vi "ARCO Main Server.vi"() -> ()   [LabVIEW 2017]
uses:
  <vilib>/OPCUA/controls/Data Type.ctl
  <vilib>/OPCUA/controls/Supported Security Policies.ctl
  <vilib>/OPCUA/server/Read Bool Array.vi
  <vilib>/OPCUA/NI OPC UA Server.lvlib
  <vilib>/OPCUA/NI OPC UA Utility.lvlib
panel:
  out "BoP Output Node":string
  out "BoP Input Node":string
  out "Result Boolean Control Node":string
  out "Result Numeric Control Node":string
  out "Result Data Node":string
  out "Spoof Boolean Control Node":string
  out "Spoof Numeric Control Node":string
  out "Spoof Data Node":string
  out "Chat Node":string
  out "Boolean Control Action Node":string
  out "Numeric Control Action Node":string
  out "certificate path 2":path
  out "certificate path":path
  out "error out":errorcluster
  out "CIET Data Node":string
  out "server endpoint URL":string
  in  "Stop":bool
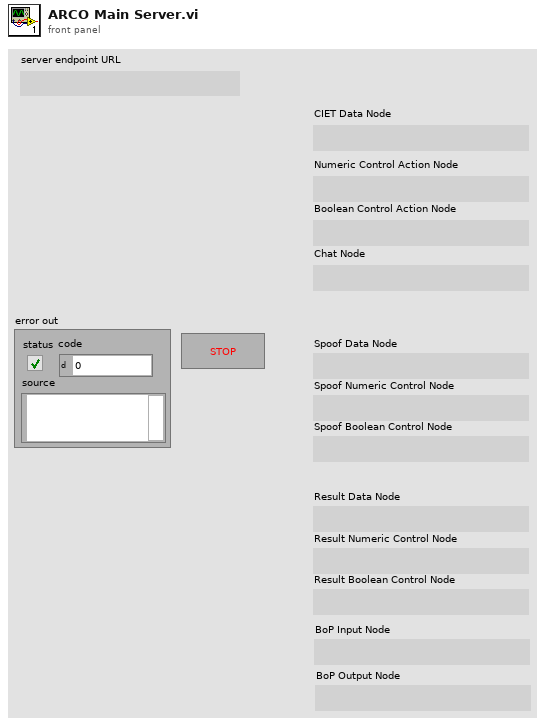
[diagram p1: front panel]
types:
  T1 = typedef "Data Type.ctl" = u16
  T2 = cluster{"name":string, "data type":T1, "access level":u16, "description":string}
  T3 = cluster{"name":string, "data type":T1, "access level 2":u16, "description":string}
  T4 = typedef "Supported Security Policies.ctl" = cluster{"None":bool, "Sign with Basic128Rsa15":bool, "Sign and Encrypt with Basic128Rsa15":bool, "Sign with Basic256":bool, "Sign and Encrypt with Basic256":bool}
  T5 = typedef "OPC UA Server Refnum.ctl" = refnum<k21>
  T6 = typedef "NodeId.ctl" = string
  T7 = cluster{"value[0]":bool, "value[1]":bool, "value[2]":bool, "value[3]":bool, "value[4]":bool, "value[5]":bool, "value[6]":bool, "value[7]":bool, "value[8]":bool}
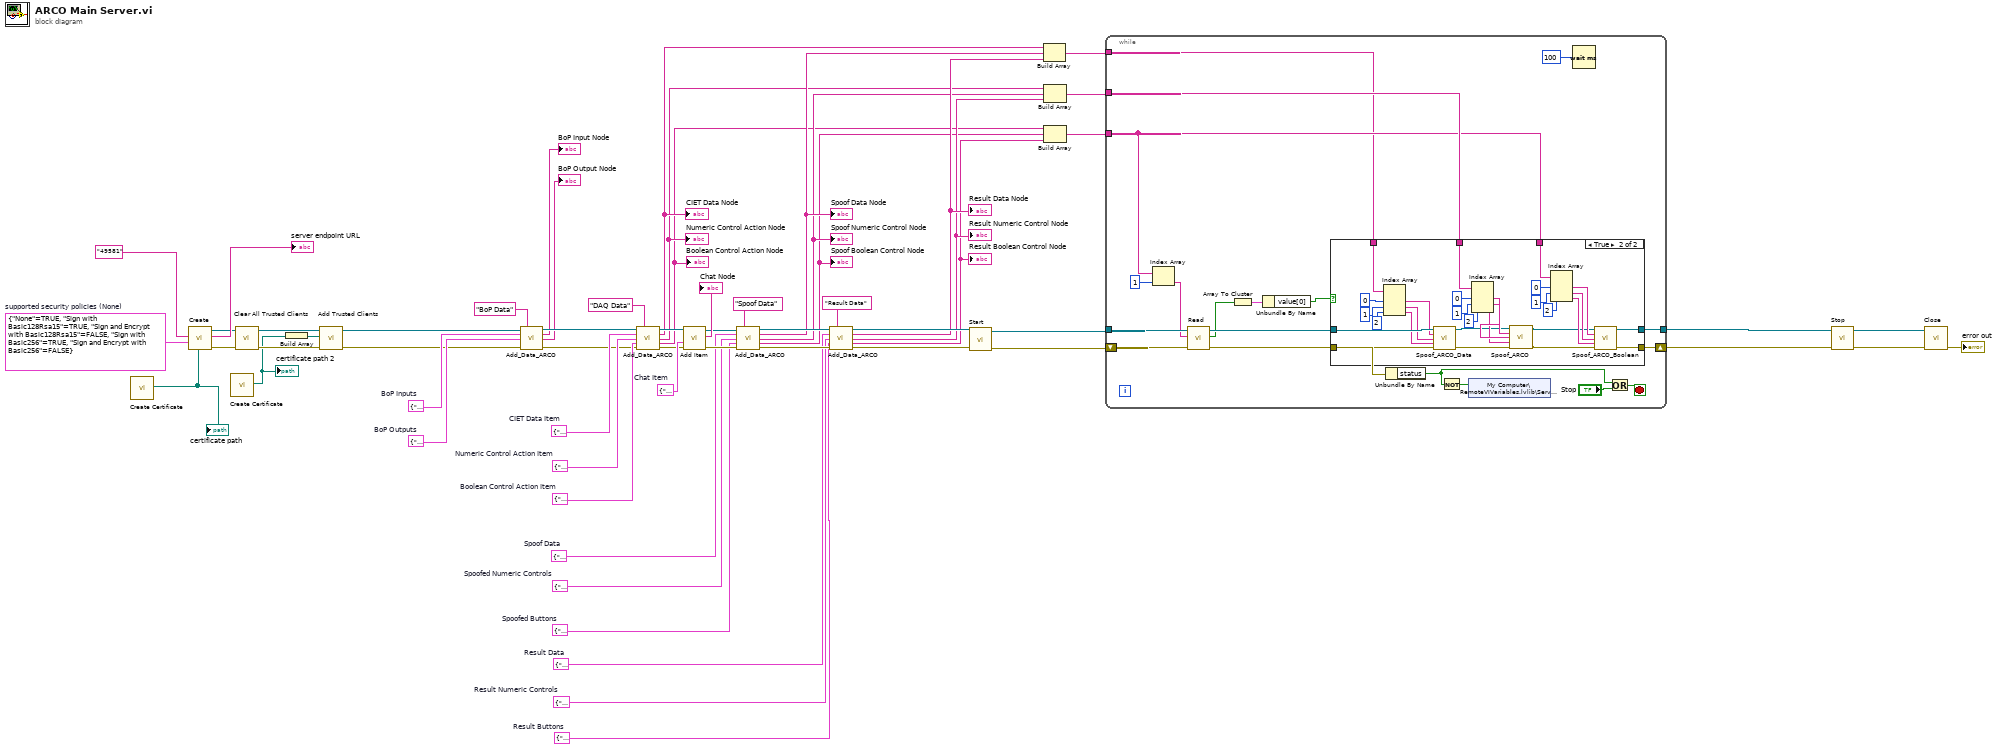
[diagram p0: block diagram]
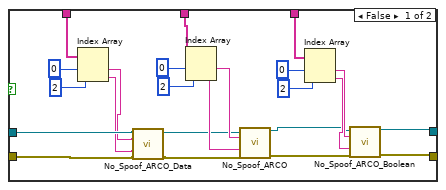
[diagram p2: hidden frame]
diagram:
  w7 = T2 {"name"="BoP Outputs", "data type"=111, "access level"=3, "description"="BoP Output Values"}  # BoP Outputs
  w8 = T2 {"name"="BoP Inputs", "data type"=111, "access level"=3, "description"="BoP Input Values"}  # BoP Inputs
  w25 = T2 {"name"="Spoofed Numeric Controls", "data type"=111, "access level"=3, "description"="Spoofed Setpoints"}  # Spoofed Numeric Controls
  w26 = T2 {"name"="Spoofed CIET Data", "data type"=111, "access level"=3, "description"="Spoofed CIET TC and FM"}  # Spoof Data
  w31 = T2 {"name"="Result Boolean Controls", "data type"=101, "access level"=3, "description"="Result Buttons"}  # Result Buttons
  w32 = T2 {"name"="Result Numeric Controls", "data type"=111, "access level"=3, "description"="Result Setpoints"}  # Result Numeric Controls
  w33 = T3 {"name"="Result CIET Data", "data type"=111, "access level 2"=3, "description"="Result CIET TC and FM"}  # Result Data
  w24 = T2 {"name"="Spoofed Boolean Controls", "data type"=101, "access level"=3, "description"="Spoofed Buttons"}  # Spoofed Buttons
  w45 = T2 {"name"="Chat", "data type"=12, "access level"=3, "description"="Chat"}  # Chat Item
  w41 = T2 {"name"="Boolean Control Actions", "data type"=101, "access level"=3, "description"="Buttons"}  # Boolean Control Action Item
  w42 = T2 {"name"="Numeric Control Actions", "data type"=111, "access level"=3, "description"="Setpoints"}  # Numeric Control Action Item
  w54 = T4 {"None"=TRUE, "Sign with Basic128Rsa15"=TRUE, "Sign and Encrypt with Basic128Rsa15"=FALSE, "Sign with Basic256"=TRUE, "Sign and Encrypt with Basic256"=FALSE}  # supported security policies (None)
  w43 = T2 {"name"="CIET Data", "data type"=111, "access level"=3, "description"="CIET TC and FM"}  # CIET Data Item
  n1 = call <vilib>:"Create Certificate.vi"() -> ("certificate path"=w49:path)  [unwired: 8 in, 3 out]
  "certificate path" <- w49
  n2 = call <vilib>:"Create.vi"("server certificate file"=w49, "supported security policies (None)"=w54, "TCP port (49580)"="49581") -> ("error out"=w50:errorcluster, "server endpoint URL"=→"server endpoint URL":string, "OPC UA server refnum out"=w51:T5)  [unwired: 6 in]
  n3 = call <vilib>:"Create Certificate.vi"() -> ("certificate path"=w48:path)  [unwired: 8 in, 3 out]
  "certificate path 2" <- w48
  n4 = call <vilib>:"Clear All Trusted Clients.vi"("error in (no error)"=w50, "OPC UA server refnum in"=w51) -> ("error out"=w52:errorcluster, "OPC UA server refnum out"=w53:T5)  [unwired: 8 in]
  n5 = Build Array(w48) -> (w47:path[])
  n6 = call <vilib>:"Add Trusted Clients.vi"("error in (no error)"=w52, "trusted client certificates"=w47, "OPC UA server refnum in"=w53) -> ("error out"=w5:errorcluster, "OPC UA server refnum out"=w6:T5)  [unwired: 7 in]
  n7 = call "Add_Data_ARCO.vi"("Refnum in"=w6, "folder name"="BoP Data", "item 1"=w8, "item 2"=w7, "error in (no error)"=w5) -> ("Refnum out"=w3:T5, "item node ID 1"=→"BoP Input Node":string, "item node ID 2"=→"BoP Output Node":string, "error out"=w4:errorcluster)  [unwired: 6 in, 1 out]
  n8 = call "Add_Data_ARCO.vi"("Refnum in"=w3, "folder name"="DAQ Data", "item 1"=w43, "item 2"=w42, "item 3"=w41, "error in (no error)"=w4) -> ("Refnum out"=w40:T5, "item node ID 1"=w20:string, "item node ID 2"=w17:string, "item node ID 3"=w14:string, "error out"=w39:errorcluster)  [unwired: 5 in]
  "CIET Data Node" <- w20
  "Numeric Control Action Node" <- w17
  "Boolean Control Action Node" <- w14
  n9 = call <vilib>:"Add Item.vi"("error in (no error)"=w39, "item"=w45, "OPC UA server refnum in"=w40) -> ("error out"=w36:errorcluster, "item node ID"=→"Chat Node":T6, "OPC UA server refnum out"=w37:T5)  [unwired: 4 in, 1 out]
  n10 = call "Add_Data_ARCO.vi"("Refnum in"=w37, "folder name"="Spoof Data", "item 1"=w26, "item 2"=w25, "item 3"=w24, "error in (no error)"=w36) -> ("Refnum out"=w34:T5, "item node ID 1"=w19:string, "item node ID 2"=w16:string, "item node ID 3"=w13:string, "error out"=w35:errorcluster)  [unwired: 5 in]
  "Spoof Data Node" <- w19
  "Spoof Numeric Control Node" <- w16
  "Spoof Boolean Control Node" <- w13
  n11 = call "Add_Data_ARCO.vi"("Refnum in"=w34, "folder name"="Result Data", "item 1"=w33, "item 2"=w32, "item 3"=w31, "error in (no error)"=w35) -> ("Refnum out"=w27:T5, "item node ID 1"=w18:string, "item node ID 2"=w15:string, "item node ID 3"=w12:string, "error out"=w28:errorcluster)  [unwired: 5 in]
  "Result Data Node" <- w18
  "Result Numeric Control Node" <- w15
  "Result Boolean Control Node" <- w12
  n12 = call <vilib>:"Start.vi"("error in (no error)"=w28, "OPC UA server refnum in"=w27) -> ("error out"=w11:errorcluster, "OPC UA server refnum out"=w59:T5)  [unwired: 7 in, 1 out]
  n13 = Build Array(w20, w19, w18) -> (w23:string[])
  n14 = Build Array(w17, w16, w15) -> (w22:string[])
  n15 = Build Array(w14, w13, w12) -> (w21:string[])
  n16 = while {
    tunnel: [w78] -> w58
    tunnel: w59 -> [w71]
    tunnel: w23 -> [w61]
    tunnel: w22 -> [w67]
    tunnel: w21 -> [w62]
    shift-right: [w76] -> w10
    shift-left: w11 -> [w72]
    stop <- w75 stop-if-true
    n17 = Index Array(array=w62, index=1) -> (element=w66:string)
    n18 = call-poly <vilib>:"Read.vi"("error in (no error)"=w72, "node ID"=w66, "OPC UA server refnum in"=w71) -> ("error out"=w69:errorcluster, "value"=w65:bool[], "OPC UA server refnum out"=w70:T5)  [unwired: 4 in, 2 out]
    n19 = Array To Cluster(array=w65) -> (cluster=w64:T7)
    n20 = Unbundle By Name(w64) -> ("value[0]"=w63:bool)
    n21 = case shown="True" w63 {
      tunnel: [w88 w131] -> w78
      tunnel: w70 -> [w82 w106]
      tunnel: w67 -> [w91 w118]
      tunnel: w62 -> [w96 w117]
      tunnel: [w87 w116] -> w76
      tunnel: w69 -> [w83 w107]
      tunnel: w61 -> [w86 w110]
      frame False {
        n22 = Index Array(array=w86, index #1=0, index #2=2 ("index")) -> (element #1=w81:string, element #2=w80:string)
        n23 = call "No_Spoof_ARCO_Data.vi"("OPC UA server refnum in"=w82, "DAQ Node"=w81, "Result Node"=w80, "error in (no error)"=w83) -> ("OPC UA server refnum out"=w85:T5, "error out"=w84:errorcluster)  [unwired: 10 in]
        n24 = Index Array(array=w91, index #1=0, index #2=2 ("index")) -> (element #1=w93:string, element #2=w92:string)
        n25 = call "No_Spoof_ARCO.vi"("OPC UA server refnum in"=w85, "DAQ Node"=w93, "Result Node"=w92, "error in (no error)"=w84) -> ("OPC UA server refnum out"=w90:T5, "error out"=w89:errorcluster)  [unwired: 10 in]
        n26 = Index Array(array=w96, index #1=0, index #2=2 ("index")) -> (element #1=w98:string, element #2=w97:string)
        n27 = call "No_Spoof_ARCO_Boolean.vi"("OPC UA server refnum in"=w90, "DAQ Node"=w98, "Result Node"=w97, "error in (no error)"=w89) -> ("OPC UA server refnum out"=w88:T5, "error out"=w87:errorcluster)  [unwired: 10 in]
      }
      frame True {
        n28 = Index Array(array=w110, index #1=0, index #2=1, index #3=2) -> (element #1=w103:string, element #2=w104:string, element #3=w105:string)
        n29 = call "Spoof_ARCO_Data.vi"("OPC UA server refnum in"=w106, "DAQ Node"=w103, "Spoof Node"=w104, "Result Node"=w105, "error in (no error)"=w107) -> ("OPC UA server refnum out"=w109:T5, "error out"=w108:errorcluster)  [unwired: 9 in]
        n30 = Index Array(array=w118, index #1=0, index #2=1, index #3=2) -> (element #1=w115:string, element #2=w114:string, element #3=w113:string)
        n31 = call "Spoof_ARCO.vi"("OPC UA server refnum in"=w109, "DAQ Node"=w115, "Spoof Node"=w114, "Result Node"=w113, "error in (no error)"=w108) -> ("OPC UA server refnum out"=w112:T5, "error out"=w111:errorcluster)  [unwired: 9 in]
        n32 = Index Array(array=w117, index #1=0, index #2=1, index #3=2) -> (element #1=w119:string, element #2=w120:string, element #3=w121:string)
        n33 = call "Spoof_ARCO_Boolean.vi"("OPC UA server refnum in"=w112, "DAQ Node"=w119, "Spoof Node"=w120, "Result Node"=w121, "error in (no error)"=w111) -> ("OPC UA server refnum out"=w131:T5, "error out"=w116:errorcluster)  [unwired: 9 in]
      }
    }
    n34 = Unbundle By Name(w69) -> ("status"=w73:bool)
    n35 = Not(x=w73) -> (.not. x?=w77:bool)
    n36 = shared-variable "My Computer\\RemoteVIVariables.lvlib\\Server Status"(w77) -> ()  [unwired: 1 in, 1 out]
    n37 = Wait (ms)(milliseconds to wait=u32 100) -> ()  [unwired: 1 out]
    n38 = Or(x=w73, y="Stop") -> (x .or. y?=w75:bool)
  }
  n39 = call <vilib>:"Stop.vi"("error in (no error)"=w10, "OPC UA server refnum in"=w58) -> ("error out"=w56:errorcluster, "OPC UA server refnum out"=w57:T5)  [unwired: 8 in]
  n40 = call <vilib>:"Close.vi"("error in (no error)"=w56, "OPC UA server refnum in"=w57) -> ("error out"=→"error out":errorcluster)  [unwired: 9 in]
